vi "get hdu names.vi"() -> ()   [LabVIEW 2023]
uses:
  gfitsio.lvlib
  cfitsio-bitpix.ctl
  gfitsio-write-image-subset-dbl-scalar.vi
panel:
  in  "file path (dialog if empty)":path=path "C:/OCI/OCI python/test23.fits"
  out "hdu name":string
  out "hdu names":string[](array[string])=["Primary", ""]
  out "hdu name (dialog if empty)":string
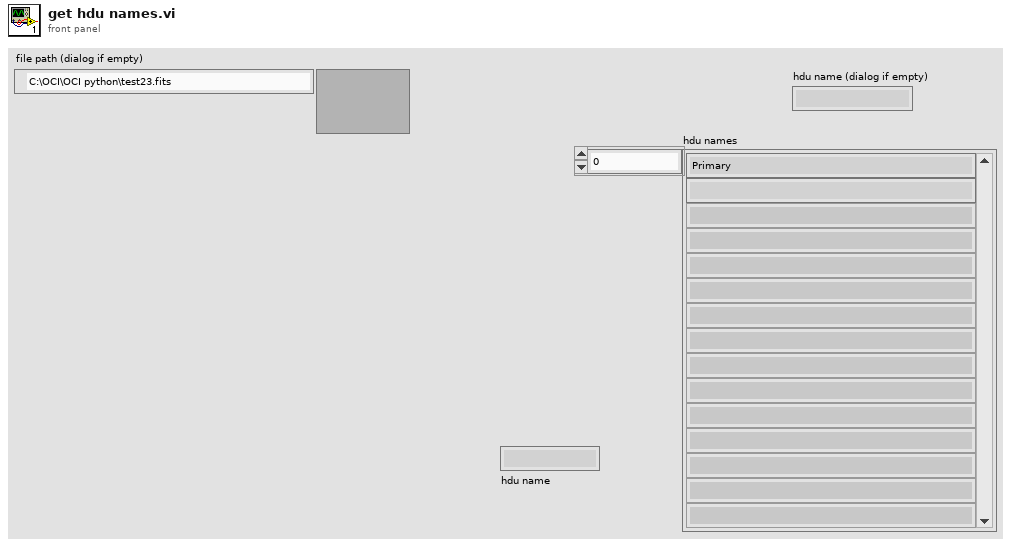
[diagram p1: front panel]
types:
  T1 = enum16{"open", "open or create", "create or replace", "create", "open (read only)"}
  T2 = typedef "gfitsio.lvlib/gfitsio-refnum.ctl" = refnum<k1>
  T3 = enum16{"open", "open or create", "create", "create or replace"}
  T4 = typedef "gfitsio.lvlib/cfitsio-bitpix.ctl" = i32
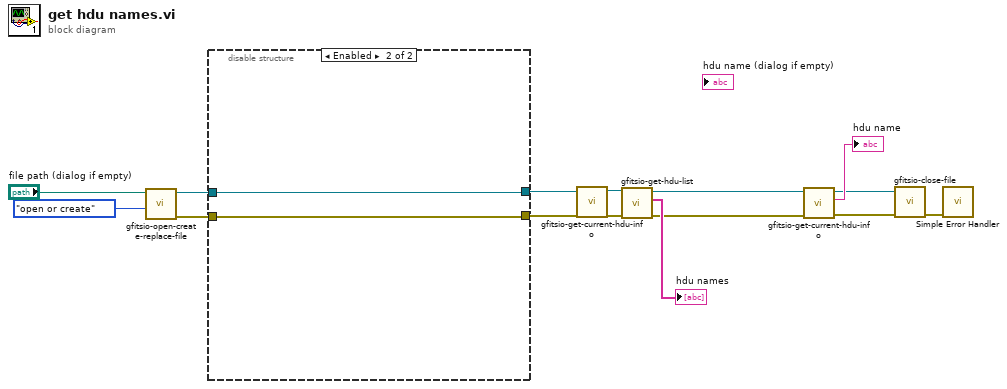
[diagram p0: block diagram]
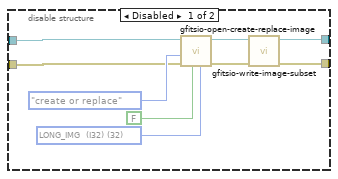
[diagram p2: hidden frame]
diagram:
  n1 = call "gfitsio-open-create-replace-file.vi"("function (open)"=T1."open or create", "file path (dialog if empty)"="file path (dialog if empty)") -> ("error out"=w5:errorcluster, "gfits refnum"=w4:T2)  [unwired: 7 in, 1 out]
  n2 = disable-structure shown="Enabled" {
    disable-tunnel: [w24 w25] -> w9
    disable-tunnel: [w23 w26] -> w8
    disable-tunnel: w5 -> [w17 w25]
    disable-tunnel: w4 -> [w16 w26]
    frame Disabled {
      w21 = T4 32 items=["<invalid type>"=0, "BYTE_IMG  (U8)"=8, "SHORT_IMG  (I16)"=16, "USHORT_IMG  (U16)"=20, "LONG_IMG  (I32)"=32, "ULONG_IMG  (U32)"=40, "FLOAT_IMG  (SGL)"=-32, "DOUBLE_IMG  (DBL)"=-64] ("image data type")
      n3 = call "gfitsio-open-create-replace-image.vi"("image data type"=w21, "advisory dialog? (display:T)"=FALSE, "error in (no error)"=w17, "function (create or replace)"=T3."create or replace" ("function (open or create)"), "gfits refnum"=w16) -> ("error out"=w18:errorcluster, "dup gfits refnum"=w19:T2)  [unwired: 4 in, 1 out]
      n4 = call-poly "gfitsio-write-image-subset.vi"("error in (no error)"=w18, "gfits refnum"=w19) -> ("error out"=w24:errorcluster, "dup gfits refnum"=w23:T2)  [unwired: 8 in]
    }
    frame Enabled {
    }
  }
  n5 = call "gfitsio-get-current-hdu-info.vi"("error in (no error)"=w9, "gfits refnum"=w8) -> ("error out"=w11:errorcluster, "dup gfits refnum"=w10:T2)  [unwired: 5 in, 3 out]
  n6 = call "gfitsio-get-hdu-list.vi"("error in (no error)"=w11, "gfits refnum"=w10) -> ("error out"=w1:errorcluster, "hdu names"=→"hdu names":string[], "dup gfits refnum"=w2:T2)  [unwired: 6 in, 1 out]
  n7 = call "gfitsio-get-current-hdu-info.vi"("error in (no error)"=w1, "gfits refnum"=w2) -> ("error out"=w13:errorcluster, "hdu name"=→"hdu name":string, "dup gfits refnum"=w12:T2)  [unwired: 5 in, 2 out]
  n8 = call "gfitsio-close-file.vi"("error in (no error)"=w13, "gfits refnum"=w12) -> ("error out"=w7:errorcluster)  [unwired: 8 in, 1 out]
  n9 = call <vilib>:"Simple Error Handler.vi"("error in (no error)"=w7) -> ()  [unwired: 4 in, 5 out]
